vi "Color Sensor Copy.vi"() -> ()   [LabVIEW 2019]
uses:
  <vilib>/Rock Robotics/SystemInterfaces/i2clib/i2c_bus.ctl
  <vilib>/Rock Robotics/WPI/MotorControl/WPI_MotorControlOpen TalonSRX.vi
  <vilib>/Rock Robotics/SystemInterfaces/DIO/FPGA_DIOPWMChannel.ctl
  Sub Systems/Control Panel Global.vi
panel:
  out "Color 3":u32(colorbox)
  out "Normalized Color":cluster{"R":dbl, "G":dbl, "B":dbl}
  out "Color 2":bool
  in  "Output":dbl
  out "Color":dbl
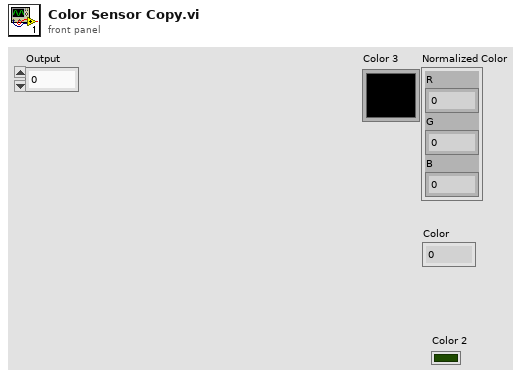
[diagram p1: front panel]
types:
  T1 = typedef "FPGA_DIOPWMChannel.ctl" = enum8{"PWM 0", "PWM 1", "PWM 2", "PWM 3", "PWM 4", "PWM 5", "PWM 6", "PWM 7", "PWM 8", "PWM 9", "PWM MXP 0", "PWM MXP 1", "PWM MXP 2", "PWM MXP 3", "PWM MXP 4", "PWM MXP 5", "PWM MXP 6", "PWM MXP 7", "PWM MXP 8", "PWM MXP 9", "Invalid"}
  T2 = typedef "i2c_bus.ctl" = enum16{"I2C On-Board", "I2C MXP", "Invalid"}
  T3 = typedef "WPI_MotorControlDeviceRef.ctl" = cluster{"DeviceStatus":errorcluster, "Type":T4, "PWM":cluster{"PWM Channel":T1, "DeadBand":T5}, "CAN":cluster{"Device Number":u8, "SetOutput VI Ref":variant, "GetOutput VI Ref":variant, "Enable VI Ref":variant, "Disable VI Ref":variant, "Data":variant}, "Invert":bool, "DIO PWM":cluster{"PWM \"Enable\" Channel":T1, "DIOChannel":T6, "PWM Rate":dbl}}
  T4 = typedef "WPI_MotorControlType.ctl" = enum16{"PWM", "CAN", "DIO PWM"}
  T5 = typedef "WPI_PWMDeadband.ctl" = cluster{"Name":string, "maxPositivePwm":i32, "minPositivePwm":i32, "centerPwm":i32, "maxNegativePwm":i32, "minNegativePwm":i32, "angularRange":u16}
  T6 = typedef "FPGA_DIOChannel.ctl" = enum8{"DIO 0", "DIO 1", "DIO 2", "DIO 3", "DIO 4", "DIO 5", "DIO 6", "DIO 7", "DIO 8", "DIO 9", "DIO MXP 0", "DIO MXP 1", "DIO MXP 2", "DIO MXP 3", "DIO MXP 4", "DIO MXP 5", "DIO MXP 6", "DIO MXP 7", "DIO MXP 8", "DIO MXP 9", "DIO MXP 10", "DIO MXP 11", "DIO MXP 12", "DIO MXP 13", "DIO MXP 14", "DIO MXP 15", "SPI Port CS1", "SPI Port CS2", "SPI Port CS3", "SPI Port MISO", "SPI Port MOSI", "Invalid"}
  T7 = typedef "Color Sensor V3 DevRef.ctl" = cluster{"I2CDevRef":T8}
  T8 = typedef "WPI_I2CDevRef.ctl" = cluster{"DevStatus":errorcluster, "Device Address":u8, "Handle":i32, "I2C Bus":T2}
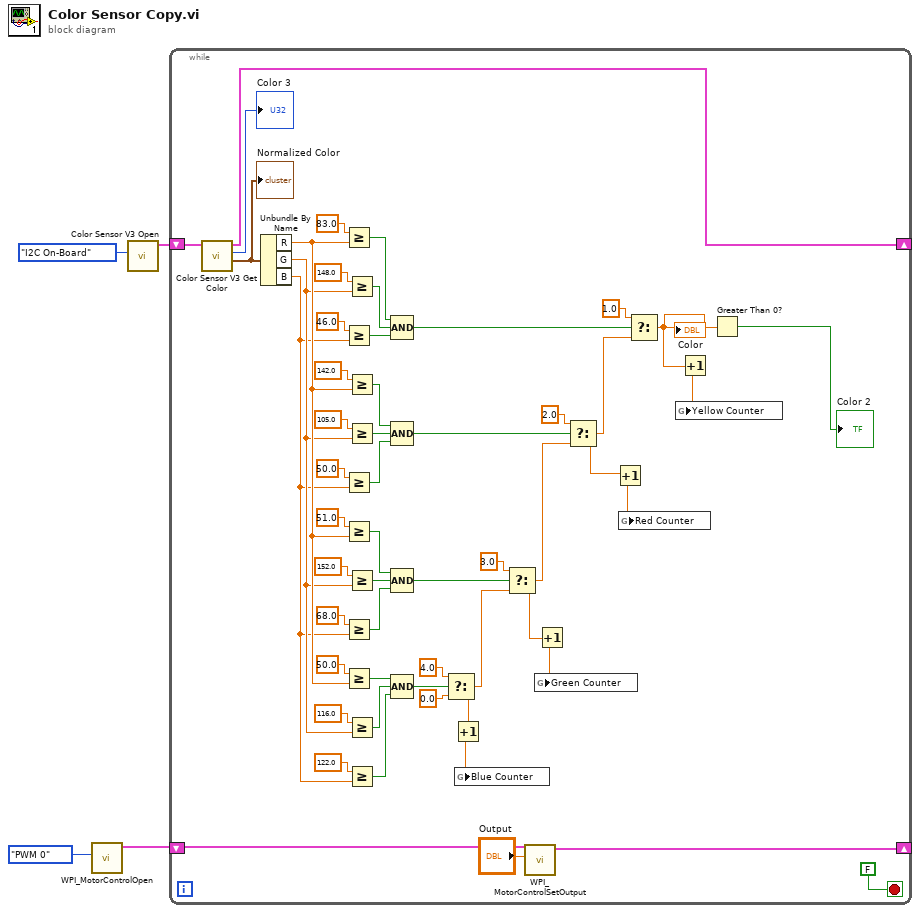
[diagram p0: block diagram]
diagram:
  n1 = call-poly <vilib>:"WPI_MotorControlOpen.vi"("PWM Channel"=FPGA_DIOPWMChannel."PWM 0") -> ("MotorControlDeviceRef"=w2:T3)  [unwired: 9 in, 1 out]
  n2 = call <vilib>:"Color Sensor V3 Open.vi"("I2C Bus"=i2c_bus."I2C On-Board") -> ("ColorSensorDevRef"=w3:T7)  [unwired: 9 in, 1 out]
  n3 = while {
    shift-right: [w56] -> _
    shift-left: w3 -> [w57]
    shift-right: [w14] -> _
    shift-left: w2 -> [w15]
    stop <- FALSE stop-if-true
    n4 = call <vilib>:"Color Sensor V3 Get Color.vi"("ColorSensorDevRef"=w57) -> ("Normalized Color"=w53:cluster{"R":dbl, "G":dbl, "B":dbl}, "Color"=→"Color 3":u32, "ColorSensorDevRef out"=w56:T7)  [unwired: 7 in, 1 out]
    "Normalized Color" <- w53
    n5 = Unbundle By Name(w53) -> ("R"=w26:dbl, "G"=w25:dbl, "B"=w24:dbl)
    n6 = Greater Or Equal?(x=83.0 ("R"), y=w26) -> (x >= y?=w45:bool)
    n7 = Greater Or Equal?(x=46.0 ("B"), y=w24) -> (x >= y?=w47:bool)
    n8 = Greater Or Equal?(x=50.0 ("B"), y=w24) -> (x >= y?=w38:bool)
    n9 = Greater Or Equal?(x=51.0 ("R"), y=w26) -> (x >= y?=w31:bool)
    n10 = Greater Or Equal?(x=68.0 ("B"), y=w24) -> (x >= y?=w33:bool)
    n11 = Greater Or Equal?(x=50.0 ("R"), y=w26) -> (x >= y?=w21:bool)
    n12 = Greater Or Equal?(x=148.0 ("G"), y=w25) -> (x >= y?=w46:bool)
    n13 = Greater Or Equal?(x=142.0 ("R"), y=w26) -> (x >= y?=w40:bool)
    n14 = Greater Or Equal?(x=105.0 ("G"), y=w25) -> (x >= y?=w39:bool)
    n15 = Greater Or Equal?(x=152.0 ("G"), y=w25) -> (x >= y?=w32:bool)
    n16 = Greater Or Equal?(x=116.0 ("G"), y=w25) -> (x >= y?=w22:bool)
    n17 = Greater Or Equal?(x=122.0 ("B"), y=w24) -> (x >= y?=w23:bool)
    n18 = Compound Arithmetic op=AND(w45, w46, w47) -> (w44:bool)
    n19 = Compound Arithmetic op=AND(w40, w39, w38) -> (w37:bool)
    n20 = Compound Arithmetic op=AND(w31, w32, w33) -> (w30:bool)
    n21 = Compound Arithmetic op=AND(w21, w22, w23) -> (w20:bool)
    n22 = Select(t=4.0, s=w20, f=0.0) -> (s? t:f=w5:dbl)
    n23 = Increment(x=w5) -> (x+1=w6:dbl)
    n24 = global write "Control Panel Global.vi" "Blue Counter"(w6) -> ()
    n25 = Select(t=3.0, s=w30, f=w5) -> (s? t:f=w7:dbl)
    n26 = call <vilib>:"WPI_MotorControlSetOutput.vi"("Output"="Output", "MotorControlDevRef"=w15) -> ("MotorControlDevRef"=w14:T3)  [unwired: 7 in, 2 out]
    n27 = Increment(x=w7) -> (x+1=w8:dbl)
    n28 = global write "Control Panel Global.vi" "Green Counter"(w8) -> ()
    n29 = Select(t=2.0, s=w37, f=w7) -> (s? t:f=w9:dbl)
    n30 = Increment(x=w9) -> (x+1=w10:dbl)
    n31 = global write "Control Panel Global.vi" "Red Counter"(w10) -> ()
    n32 = Select(t=1.0, s=w44, f=w9) -> (s? t:f=w12:dbl)
    "Color" <- w12
    n33 = Increment(x=w12) -> (x+1=w11:dbl)
    n34 = global write "Control Panel Global.vi" "Yellow Counter"(w11) -> ()
    n35 = Greater Than 0?(x=w12) -> (x > 0?=→"Color 2":bool)
  }
